vi "pick up recycling bins.vi"(0 "CoPilot":refnum<k33>, 3 "Refnum in":refnum<k33>) -> (10 "Refnum out":refnum<k33>)   [LabVIEW 2014]
uses:
  TeleopCmd.ctl
  CmdFlag.ctl
  Co-Pilot_game_control.ctl
  Lifter Hights.vi
panel:
  in  "Distance":dbl=1.0 format="%#_13g"
  out "CoPilot 2":refnum<k33>
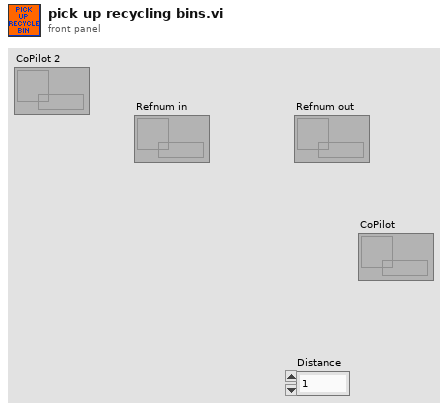
[diagram p1: front panel]
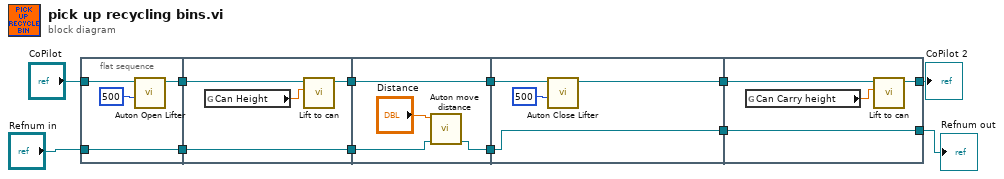
[diagram p0: block diagram]
diagram:
  n1 = flat-sequence {
    tunnel: "Refnum in" -> [w16]
    tunnel: [w16] -> w11
    tunnel: "CoPilot" -> [w15]
    tunnel: [w14] -> w9
    tunnel: w11 -> [w20]
    tunnel: [w20] -> w6
    tunnel: w9 -> [w19]
    tunnel: [w18] -> w4
    tunnel: w6 -> [w22]
    tunnel: [w21] -> w5
    tunnel: w4 -> [w24]
    tunnel: [w24] -> w3
    tunnel: [w28] -> w8
    tunnel: w3 -> [w27]
    tunnel: w5 -> [w25]
    tunnel: [w25] -> w2
    tunnel: w8 -> [w32]
    tunnel: [w31] -> w7
    tunnel: [w29] -> w1
    tunnel: w2 -> [w29]
    frame #0 {
      n2 = call "Auton Open Lifter.vi"("milliseconds to wait"=u32 500, "CoPilot"=w15) -> ("CoPilot 2"=w14:refnum<k33>)  [unwired: 9 in]
    }
    frame #1 {
      n3 = global read "Lifter Hights.vi" "Can Height"() -> (w17:dbl)
      n4 = call "Lift to can.vi"("Desired Height"=w17, "Refnum in"=w19) -> ("Refnum out"=w18:refnum<k33>)  [unwired: 7 in]
    }
    frame #2 {
      n5 = call "Auton move distance.vi"("Distance"="Distance", "Refnum in"=w22) -> ("rt fifo out"=w21:refnum<k33>)  [unwired: 7 in, 1 out]
    }
    frame #3 {
      n6 = call "Auton Close Lifter.vi"("milliseconds to wait"=u32 500, "CoPilot"=w27) -> ("CoPilot 2"=w28:refnum<k33>)  [unwired: 9 in]
    }
    frame #4 {
      n7 = global read "Lifter Hights.vi" "Can Carry height"() -> (w30:dbl)
      n8 = call "Lift to can.vi"("Desired Height"=w30, "Refnum in"=w32) -> ("Refnum out"=w31:refnum<k33>)  [unwired: 7 in]
    }
  }
  "Refnum out" <- w1
  "CoPilot 2" <- w7
